vi "Experimental Parameters Menu.vi"() -> ()   [LabVIEW 2013]
panel:
  in  "Ramp Rate (nm/ms)":dbl
  in  "Number of Samples":dbl
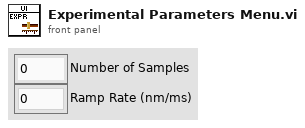
[diagram p1: front panel]
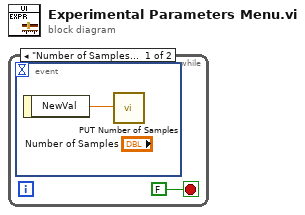
[diagram p0: block diagram]
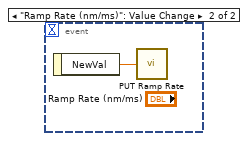
[diagram p2: hidden frame]
diagram:
  n1 = while {
    stop <- FALSE stop-if-true
    n2 = event shown="[0] \"Number of Samples\": Value Change" {
      selector: _ -> [_ _]
      dyn-events: _ -> [_ _]
      timeout: _ -> [_ _]
      event "Number of Samples": Value Change {
        n3 = event-data() -> ("NewVal"=w2:dbl)  [unwired: 1 in]
        n4 = call "PUT Number of Samples.vi"("Number of Samples"=w2) -> ()
      }
      event "Ramp Rate (nm/ms)": Value Change {
        n5 = event-data() -> ("NewVal"=w3:dbl)  [unwired: 1 in]
        n6 = call "PUT Ramp Rate.vi"("Ramp Rate"=w3) -> ()
      }
    }
  }
